vi "Etch-A-Sketch.vi"() -> ()   [LabVIEW 2017]
uses:
  Lockin/Lockin SR830.lvclass
  C:/LabVIEW-programs-dev/Instruments/Utility Classes/Readable/Readable.lvclass
  Wavelength meter/Wavelength Meter.lvclass
  Photon Counter/Photon Counter SR400.lvclass
  DAQ/DAQmx Analog.lvclass
  Power Meter/Power Meter.lvclass
  Fluke Multimeter/Fluke Multimeter.lvclass
  Cryostat/Cryostat.lvclass
  Utility Classes/Collection/Collection.lvclass
  <vilib>/Utility/file.llb/Write To Spreadsheet File (DBL).vi
  Main/Global/Misc.vi
  Main/Global/Flags.vi
  File IO/File IO.lvclass
  <vilib>/Analysis/NI_AALBase.lvlib
  Utility Classes/Readable/Readable.lvclass
panel:
  in  "Cryostat \nTemperature":bool
  in  "Fluke":bool
  out "Ave/Std Dev":dbl[](array[numeric])
  out "Average":dbl[](array[numeric])
  in  "Reset\nGraph":bool
  out "Y Range Extreme Value":dbl format="%#_4g"
  out "Latest Points":dbl[](array[numeric]) format="%#_5g"
  in  "Comments":string
  in  "Power Meter":bool
  out "Update Legend":bool
  in  "# of Points":i32=50 caption="Enter how many points to\nuse for Ave & Std Dev"
  out "Standard\nDeviation":dbl[](array[numeric])
  in  "Lockin \nSR810":bool
  in  "Lockin \nSR830":bool
  in  "Analog":bool
  in  "Photon \nCounter":bool
  in  "Wavelength \nMeter":bool
  in  "Graph Toggle":bool[](array[boolean])=[FALSE, FALSE, FALSE, FALSE, FALSE, FALSE, FALSE, FALSE, FALSE]
  in  "Display last":dbl[unit]=10.0
  in  "Time per point (s)":dbl[unit]=0.05 min=0.01 max=10.0
  in  "Start/Stop":bool
  out "XY Graph":T1(graph)
  in  "savedata?":bool
  in  "File Name":path
  in  "endprgm":bool
  # "<-- Select which instruments to use"
  # "Etch-A-Sketch"
  # "Don't\nSave"
  # "Save"
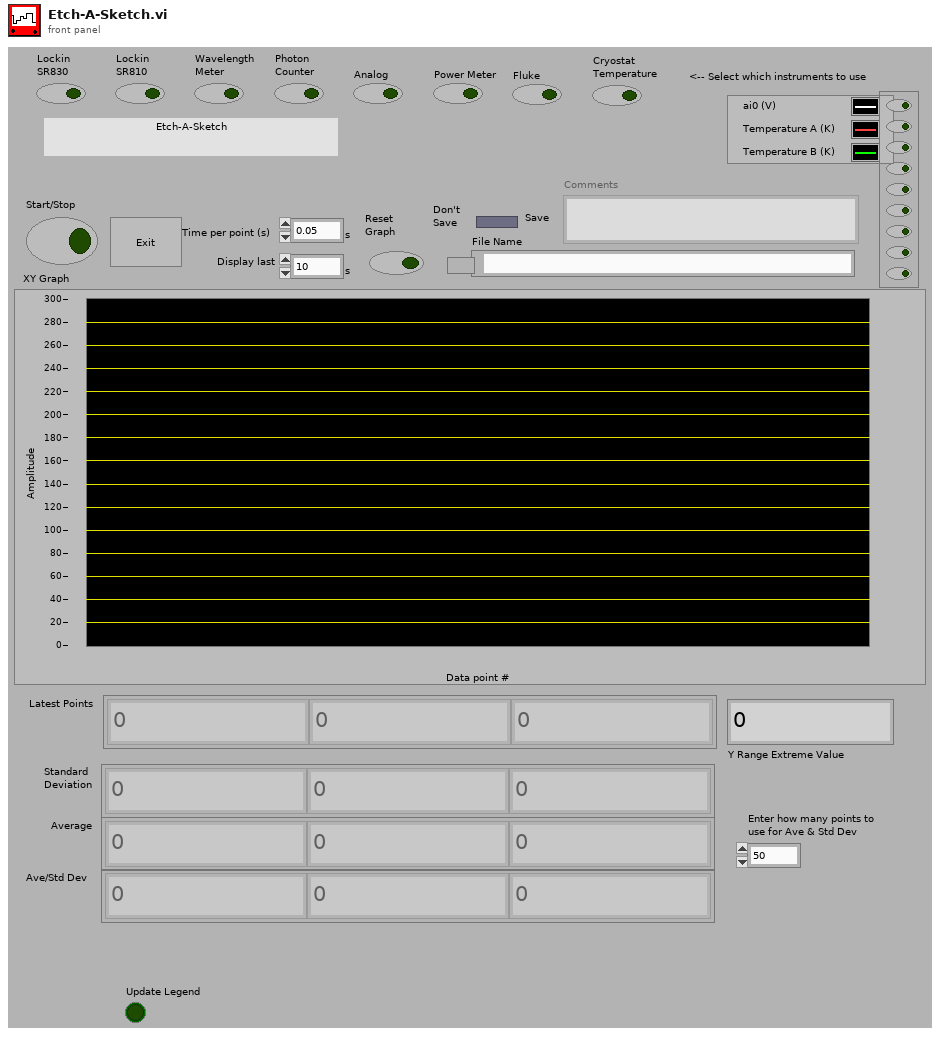
[diagram p1: front panel]
types:
  T1 = cluster{"Data Points":cluster{"t":timestamp, "x":dbl}[]}[]
  T2 = enum16{"open", "replace", "create", "open or create", "replace or create", "replace or create with confirmation"}
  T3 = typedef "Readable.lvclass/TX Graph.ctl" = cluster{"Data Points":cluster{"t":timestamp, "x":dbl}[]}[]
  T4 = typedef "Readable.lvclass/Channel Units.ctl" = string[]
  T5 = typedef "Readable.lvclass/Channel Names.ctl" = string[]
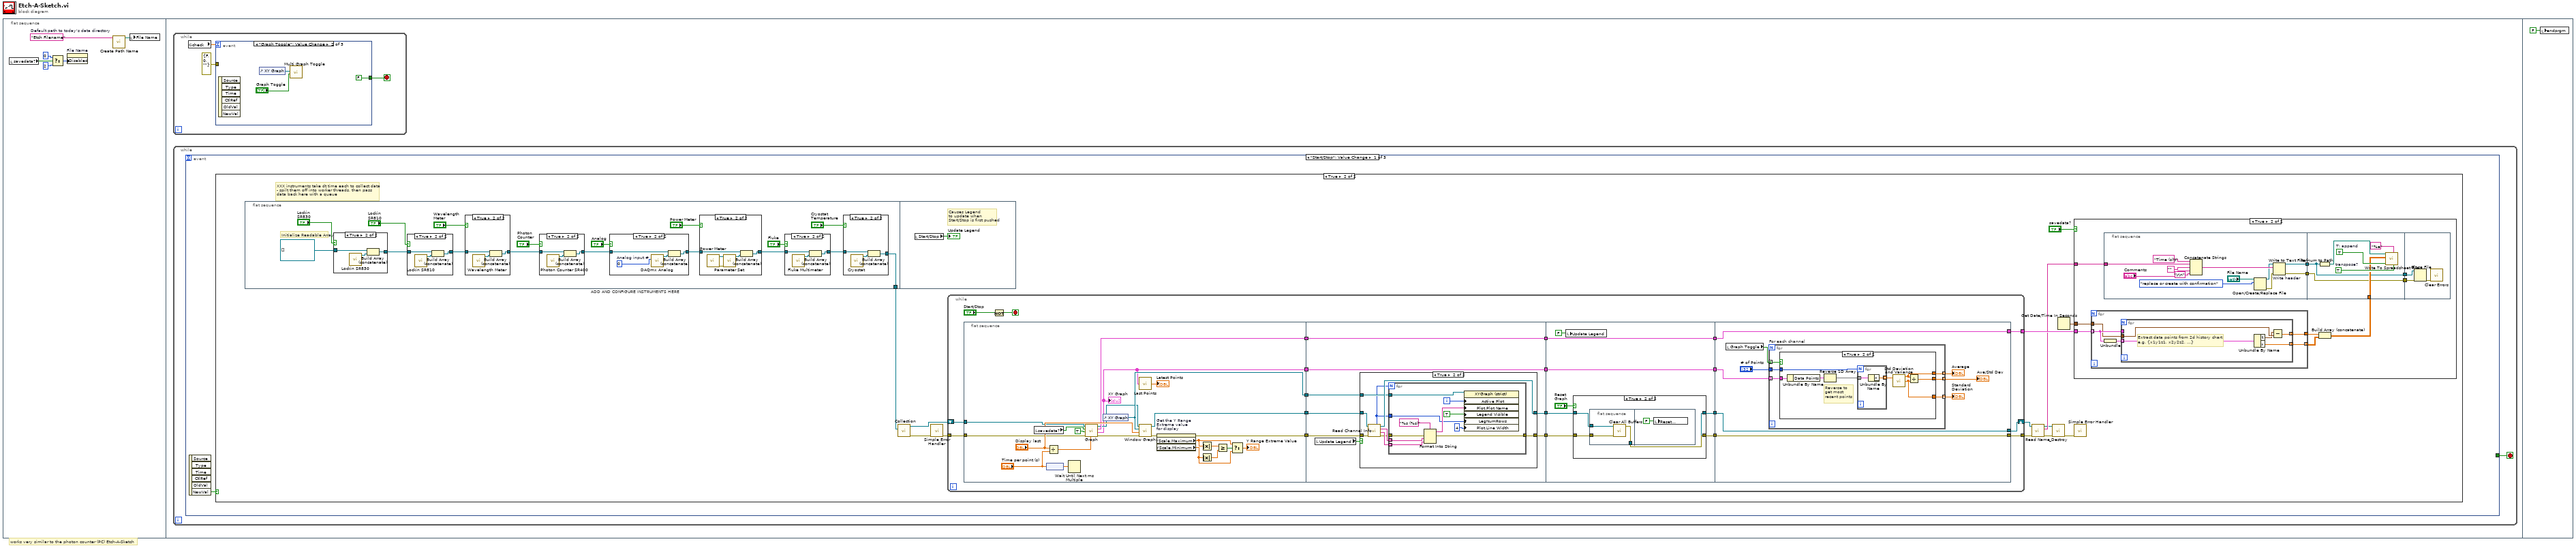
[diagram p0: block diagram]
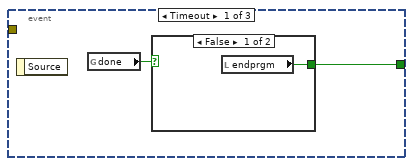
[diagram p2: hidden frame]
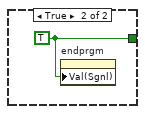
[diagram p3: hidden frame]
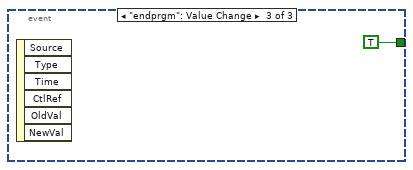
[diagram p4: hidden frame]
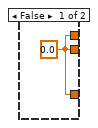
[diagram p9: hidden frame]
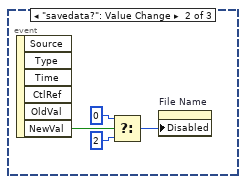
[diagram p18: hidden frame]
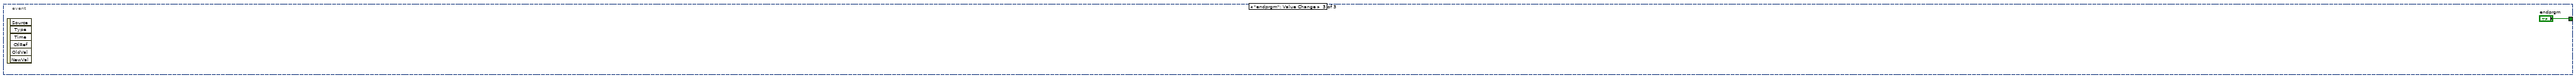
[diagram p19: hidden frame]
diagram:
  # "works very similar to the photon counter (PC) Etch-A-Sketch"
  n1 = flat-sequence {
    frame #0 {
      w1 = "Etch Filename"  # Default path to today's data directory
      n2 = local read "savedata?"() -> (w4:bool)
      n3 = Select(t=0, s=w4, f=2) -> (s? t:f=w3:i32)
      n4 = property on="File Name" class="Path"("Disabled"=w3) -> ()  [unwired: 2 in, 2 out]
      n5 = call "Create Path Name.vi"("filename"=w1) -> ("path"=w2:path)  [unwired: 1 in, 5 out]
      n6 = local write "File Name"(w2) -> ()
    }
    frame #1 {
      n7 = while {
        stop <- w9 stop-if-true
        n8 = global read "Misc.vi" "check"() -> (w8:dbl)
        n9 = event shown="[1] \"Graph Toggle\": Value Change" {
          selector: _ -> [_ _ _]
          dyn-events: _ -> [_ _ _]
          timeout: w8 -> [_ _ _]
          tunnel: [w10 FALSE TRUE] -> w9
          tunnel: errorcluster {"status"=FALSE, "code"=0, "source"=""} ("error out") -> [_ _ _]
          event Timeout {
            n10 = event-data() -> ()  [unwired: 2 out]
            n11 = global read "Flags.vi" "done"() -> (w11:bool)
            n12 = case shown="False" w11 {
              tunnel: [w12 w13] -> w10
              frame False {
                n13 = local read "endprgm"() -> (w12:bool)
              }
              frame True {
                w13 = TRUE
                n14 = property on="endprgm" class="Bool (strict)"("Val(Sgnl)"=w13) -> ()  [unwired: 2 in, 2 out]
              }
            }
          }
          event "Graph Toggle": Value Change {
            n15 = event-data() -> ()  [unwired: 7 out]
            n16 = control-ref of="XY Graph"() -> (w16:refnum<vi>)
            n17 = call "Multi Graph Toggle.vi"("Array"="Graph Toggle", "Waveform Chart"=w16) -> ()  [unwired: 1 in, 9 out]
          }
          event "endprgm": Value Change {
            n18 = event-data() -> ()  [unwired: 7 out]
          }
        }
      }
      n19 = while {
        stop <- w18 stop-if-true
        n20 = event shown="[0] \"Start/Stop\": Value Change" {
          selector: _ -> [_ _ _]
          dyn-events: _ -> [_ _ _]
          timeout: _ -> [_ _ _]
          tunnel: [_ _ "endprgm"] -> w18
          event "Start/Stop": Value Change {
            n21 = event-data() -> ("NewVal"=w19:bool)  [unwired: 6 out]
            n22 = case shown="True" w19 {
              frame False {
              }
              frame True {
                # "XXX instruments take dt time each to collect data\n- spilt them off into worker threads, then pass\ndata back here with a queue"
                n23 = flat-sequence "ADD AND CONFIGURE INSTRUMENTS HERE" {
                  tunnel: [w194] -> w20
                  frame #0 {
                    # "Initialize Readable Array"
                    n24 = case shown="True" "Lockin \nSR830" {
                      tunnel: refnum<class "Lockin SR830.lvclass">[] [] ("appended array") -> [w228 w230]
                      tunnel: [w228 w229] -> w206
                      frame False {
                      }
                      frame True {
                        n25 = call "Lockin SR830.vi"() -> ("Lockin SR830 out"=w231:refnum<class "Lockin SR830.lvclass">)  [unwired: 10 in, 1 out]
                        n26 = Build Array (concatenate)(w230, w231) -> (w229:refnum<class "Lockin SR830.lvclass">[])
                      }
                    }
                    n27 = case shown="True" "Lockin \nSR810" {
                      tunnel: w206 -> [w224 w227]
                      tunnel: [w224 w225] -> w205
                      frame False {
                      }
                      frame True {
                        n28 = call "Lockin SR810.vi"() -> ("Lockin SR830 out"=w226:refnum<class "Lockin SR830.lvclass">)  [unwired: 10 in, 1 out]
                        n29 = Build Array (concatenate)(w227, w226) -> (w225:refnum<class "Lockin SR830.lvclass">[])
                      }
                    }
                    n30 = case shown="True" "Wavelength \nMeter" {
                      tunnel: [w232 w234] -> w208
                      tunnel: w205 -> [w232 w233]
                      frame False {
                      }
                      frame True {
                        n31 = call "Wavelength Meter.vi"() -> ("Wavelength Meter out"=w235:refnum<class "Wavelength Meter.lvclass">)  [unwired: 1 in, 10 out]
                        n32 = Build Array (concatenate)(w233, w235) -> (w234:refnum<class "Readable.lvclass">[])
                      }
                    }
                    n33 = case shown="True" "Photon \nCounter" {
                      tunnel: [w236 w238] -> w209
                      tunnel: w208 -> [w236 w237]
                      frame False {
                      }
                      frame True {
                        n34 = call "Photon Counter SR400.vi"() -> ("Photon Counter SR400 out"=w239:refnum<class "Photon Counter SR400.lvclass">)  [unwired: 3 in, 8 out]
                        n35 = Build Array (concatenate)(w237, w239) -> (w238:refnum<class "Readable.lvclass">[])
                      }
                    }
                    n36 = case shown="True" "Analog" {
                      tunnel: w209 -> [w240 w242]
                      tunnel: [w240 w241] -> w198
                      frame False {
                      }
                      frame True {
                        w244 = u8 0  # Analog input #
                        n37 = call "DAQmx Analog.vi"("Analog input #"=w244) -> ("DAQmx Analog out"=w243:refnum<class "DAQmx Analog.lvclass">)  [unwired: 10 out]
                        n38 = Build Array (concatenate)(w242, w243) -> (w241:refnum<class "Readable.lvclass">[])
                      }
                    }
                    n39 = case shown="True" "Power Meter" {
                      tunnel: w198 -> [w218 w223]
                      tunnel: [w218 w222] -> w197
                      frame False {
                      }
                      frame True {
                        n40 = call "Power Meter.vi"() -> ("error out"=w219:errorcluster, "Power Meter out"=w221:refnum<class "Power Meter.lvclass">)  [unwired: 10 in]
                        n41 = call "Parameter Set.vi"("error in (no error)"=w219, "Power Meter in"=w221) -> ("Power Meter out"=w220:refnum<class "Power Meter.lvclass">)  [unwired: 8 in, 1 out]
                        n42 = Build Array (concatenate)(w223, w220) -> (w222:refnum<class "Readable.lvclass">[])
                      }
                    }
                    n43 = case shown="True" "Fluke" {
                      tunnel: w197 -> [w214 w217]
                      tunnel: [w214 w216] -> w195
                      frame False {
                      }
                      frame True {
                        n44 = call "Fluke Multimeter.vi"() -> ("Fluke Multimeter out"=w215:refnum<class "Fluke Multimeter.lvclass">)  [unwired: 10 in, 1 out]
                        n45 = Build Array (concatenate)(w217, w215) -> (w216:refnum<class "Readable.lvclass">[])
                      }
                    }
                    n46 = case shown="True" "Cryostat \nTemperature" {
                      tunnel: w195 -> [w210 w213]
                      tunnel: [w210 w212] -> w194
                      frame False {
                      }
                      frame True {
                        n47 = call "Cryostat.vi"() -> ("Cryostat out"=w211:refnum<class "Cryostat.lvclass">)  [unwired: 10 in, 1 out]
                        n48 = Build Array (concatenate)(w213, w211) -> (w212:refnum<class "Readable.lvclass">[])
                      }
                    }
                  }
                  frame #1 {
                    # "Causes Legend\nto update when\nStart/Stop is first pushed"
                    n49 = local read "Start/Stop"() -> (→"Update Legend":bool)
                  }
                }
                n50 = call "Collection.vi"("Array"=w20) -> ("error out"=w26:errorcluster, "Collection.lvclass out"=w27:refnum<class "Collection.lvclass">)  [unwired: 2 in, 7 out]
                n51 = call <vilib>:"Simple Error Handler.vi"("error in (no error)"=w26) -> ("error out"=w32:errorcluster)  [unwired: 1 in, 7 out]
                n52 = while {
                  shift-right: [w89] -> w31
                  shift-left: w27 -> [w91]
                  tunnel: w32 -> [w92]
                  tunnel: [w90] -> w29
                  tunnel: [w88] -> w21
                  stop <- w93 stop-if-true
                  n53 = flat-sequence {
                    tunnel: w92 -> [w112]
                    tunnel: w91 -> [w111]
                    tunnel: [w110] -> w87
                    tunnel: [w104] -> w86
                    tunnel: [w107] -> w85
                    tunnel: [w102] -> w84
                    tunnel: [w106] -> w83
                    tunnel: w87 -> [w119]
                    tunnel: [w119] -> w82
                    tunnel: w86 -> [w118]
                    tunnel: [w118] -> w81
                    tunnel: w85 -> [w125]
                    tunnel: w84 -> [w124]
                    tunnel: w83 -> [w123]
                    tunnel: [w121] -> w80
                    tunnel: [w120] -> w79
                    tunnel: w82 -> [w149]
                    tunnel: [w149] -> w78
                    tunnel: [w153] -> w77
                    tunnel: [w151] -> w76
                    tunnel: w81 -> [w148]
                    tunnel: [w148] -> w75
                    tunnel: w80 -> [w154]
                    tunnel: w79 -> [w152]
                    tunnel: [w172] -> w90
                    tunnel: w78 -> [w172]
                    tunnel: [w171] -> w89
                    tunnel: w77 -> [w171]
                    tunnel: [w170] -> w88
                    tunnel: w76 -> [w170]
                    tunnel: w75 -> [w175]
                    frame #0 {
                      n54 = local read "savedata?"() -> (w113:bool)
                      n55 = node("Time per point (s)") -> (w108:dbl)
                      n56 = Divide(x="Display last", y="Time per point (s)") -> (x/y=w115:dbl)
                      n57 = Wait Until Next ms Multiple(millisecond multiple=w108) -> ()  [unwired: 1 out]
                      n58 = call-dynamic "Graph.vi"("Ring size (points) (1024)"=w115, "error in (no error)"=w112, "Store Ring? (f)"=TRUE, "Store History? (f)"=w113, "Collection in"=w111) -> ("error out"=w116:errorcluster, "Ring Buffers"=w104:T3, "History Buffers"=w110:T3, "Collection out"=w105:refnum<class "Collection.lvclass">)  [unwired: 3 out]
                      "XY Graph" <- w104
                      n59 = control-ref of="XY Graph"() -> (w107:refnum<vi>)
                      n60 = call "Last Points.vi"("Ring Buffers"=w104) -> ("Latest Points"=→"Latest Points":dbl[])
                      n61 = call-dynamic "Window Graph.vi"("error in (no error)"=w116, "Window"="Display last", "Graph ref"=w107, "Readable in"=w105) -> ("error out"=w101:errorcluster, "Readable out"=w106:refnum<class "Collection.lvclass">)  [unwired: 6 in]
                      n62 = property on="Get the Y Range\nExtreme value\nfor display" class="XYGraph (strict)"(error in=w101) -> (error out=w102:errorcluster, "YScale.Maximum"=w97:dbl, "YScale.Minimum"=w96:dbl)  [unwired: 1 in, 1 out]
                      n63 = Absolute Value(x=w97) -> (abs(x)=w100:dbl)
                      n64 = Absolute Value(x=w96) -> (abs(x)=w99:dbl)
                      n65 = Greater Or Equal?(x=w100, y=w99) -> (x >= y?=w98:bool)
                      n66 = Select(t=w97, s=w98, f=w96) -> (s? t:f=→"Y Range Extreme Value":dbl)
                    }
                    frame #1 {
                      n67 = local read "Update Legend"() -> (w122:bool)
                      n68 = case shown="True" w122 {
                        tunnel: w123 -> [w126 w136]
                        tunnel: [w126 w135] -> w121
                        tunnel: w124 -> [w127 w132]
                        tunnel: [w127 w130] -> w120
                        tunnel: w125 -> [_ w129]
                        frame False {
                        }
                        frame True {
                          n69 = call "Read Channel Info.vi"("error in (no error)"=w132, "Readable.lvclass in"=w136) -> ("error out"=w131:errorcluster, "Channel Units"=w133:T4, "Channel Names"=w134:T5, "Readable.lvclass out"=w135:refnum<class "Collection.lvclass">, "#Channels"=w128:i32)  [unwired: 5 in]
                          n70 = for {
                            N: w128 -> [_]
                            tunnel: w134 -> [w144] mode=indexing
                            tunnel: w131 -> [w146]
                            tunnel: w133 -> [w143] mode=indexing
                            tunnel: [w141] -> w130
                            tunnel: w129 -> [w140]
                            tunnel: w128 -> [w138]
                            i -> [w147]
                            n71 = Format Into String(format string="%s (%s)", error in=w146, w144, w143) -> (resulting string=w142:string, error out=w141:errorcluster)  [unwired: 1 in]
                            n72 = property on="Property Node" class="XYGraph (strict)"(reference=w140, "Active Plot"=w147, "Plot.Plot Name"=w142, "Legend Visible"=TRUE ("Legend:Visible"), "LegNumRows"=w138, "Plot.Line Width"=u32 4 ("x")) -> ()  [unwired: 1 in, 2 out]
                          }
                        }
                      }
                    }
                    frame #2 {
                      n73 = local write "Update Legend"(FALSE ("Update Legend")) -> ()
                      n74 = case shown="True" "Reset\nGraph" {
                        tunnel: w154 -> [w157 w161]
                        tunnel: [w157 w158] -> w153
                        tunnel: w152 -> [w156 w160]
                        tunnel: [w156 w159] -> w151
                        frame False {
                        }
                        frame True {
                          n75 = flat-sequence {
                            tunnel: w161 -> [w165]
                            tunnel: w160 -> [w164]
                            tunnel: [w163] -> w159
                            tunnel: [w162] -> w158
                            frame #0 {
                              n76 = call "Clear All Buffers.vi"("error in (no error)"=w164, "Collection.lvclass In"=w165) -> ("error Out"=w163:errorcluster, "Collection.lvclass Out"=w162:refnum<class "Collection.lvclass">)  [unwired: 8 in]
                            }
                            frame #1 {
                              n77 = local write "Reset\nGraph"(FALSE ("Clear")) -> ()
                            }
                          }
                        }
                      }
                    }
                    frame #3 {
                      n78 = local read "Graph Toggle"() -> (w167:bool[])
                      n79 = for "For each channel" {
                        tunnel: w175 -> [w181] mode=indexing
                        tunnel: "# of Points" -> [w180]
                        tunnel: [w179] -> w173 mode=indexing
                        tunnel: w167 -> [w178] mode=indexing
                        tunnel: [w177] -> w169 mode=indexing
                        tunnel: [w176] -> w168 mode=indexing
                        n80 = case shown="True" w178 {
                          tunnel: w181 -> [_ w190]
                          tunnel: w180 -> [_ w187]
                          tunnel: [w182 w186] -> w179
                          tunnel: [w182 w183] -> w177
                          tunnel: [w182 w185] -> w176
                          frame False {
                            w182 = 0.0 ("standard deviation")
                          }
                          frame True {
                            # "Reverse to\nget most \nrecent points"
                            n81 = Unbundle By Name(w190) -> ("Data Points"=w189:cluster{"t":timestamp, "x":dbl}[])
                            n82 = Reverse 1D Array(array=w189) -> (reversed array=w188:cluster{"t":timestamp, "x":dbl}[])
                            n83 = for {
                              N: w187 -> [_]
                              tunnel: w188 -> [w192] mode=indexing
                              tunnel: [w191] -> w184 mode=indexing
                              n84 = Unbundle By Name(w192) -> ("x"=w191:dbl)
                            }
                            n85 = call <vilib>:"Std Deviation and Variance.vi"("X"=w184) -> ("mean"=w183:dbl, "standard deviation"=w186:dbl)  [unwired: 1 in, 1 out]
                            n86 = Divide(x=w183, y=w186) -> (x/y=w185:dbl)
                          }
                        }
                      }
                      "Standard\nDeviation" <- w173
                      "Average" <- w169
                      "Ave/Std Dev" <- w168
                    }
                  }
                  n87 = Not(x="Start/Stop") -> (.not. x?=w93:bool)
                }
                n88 = call-dynamic "Read Name.vi"("error in (no error)"=w21, "Instrument.lvclass in"=w31) -> ("error out"=w22:errorcluster, "Name"=w25:string, "Instrument.lvclass out"=w24:refnum<class "Collection.lvclass">)  [unwired: 7 out]
                n89 = call-dynamic "_Destroy.vi"("error in (no error)"=w22, "Collection in"=w24) -> ("error out"=w23:errorcluster)  [unwired: 9 out]
                n90 = Get Date/Time In Seconds() -> (seconds since 1Jan1904=w28:timestamp)
                n91 = case shown="True" "savedata?" {
                  tunnel: w25 -> [_ w38]
                  tunnel: w29 -> [_ w37]
                  tunnel: w28 -> [_ w36]
                  frame False {
                  }
                  frame True {
                    n92 = for {
                      tunnel: w37 -> [w68] mode=indexing
                      tunnel: [w69] -> w33 mode=indexing
                      tunnel: [w66] -> w35
                      tunnel: w36 -> [w65]
                      n93 = Unbundle(w68) -> ("Data Points"=w67:cluster{"t":timestamp, "x":dbl}[])
                      n94 = for {
                        tunnel: [w73] -> w69 mode=indexing
                        tunnel: w68 -> [_]
                        tunnel: w67 -> [w74] mode=indexing
                        tunnel: [w70] -> w66 mode=indexing
                        tunnel: w65 -> [w72]
                        # "Extract data points from 2d history chart \ne.g. {x1y1z1, x2y2z2, ...}"
                        n95 = Unbundle By Name(w74) -> ("t"=w71:timestamp, "x"=w73:dbl)
                        n96 = Subtract(x=w71, y=w72) -> (x-y=w70:dbl)
                      }
                    }
                    n97 = flat-sequence {
                      tunnel: [w53] -> w41
                      tunnel: [w50] -> w39
                      tunnel: w38 -> [w51]
                      tunnel: [w57] -> w42
                      tunnel: w41 -> [w57]
                      tunnel: w34 -> [w59]
                      tunnel: [w55] -> w40
                      tunnel: w39 -> [w55]
                      tunnel: w42 -> [w64]
                      tunnel: w40 -> [w63]
                      frame #0 {
                        n98 = Concatenate Strings("Time (s)\t" ("string"), w51, "", "Comments", "\r\n") -> (w48:string)
                        n99 = Open/Create/Replace File(file path (use dialog)="File Name", operation (0:open)=T2."replace or create with confirmation") -> (refnum out=w46:refnum<file>, error out=w49:errorcluster)  [unwired: 1 in, 4 out]
                        n100 = Write to Text File "Write header"(file (use dialog)=w46, text=w48, error in=w49) -> (refnum out=w53:refnum<file>, error out=w50:errorcluster)  [unwired: 2 out]
                      }
                      frame #1 {
                        w60 = TRUE  # transpose?
                        w61 = TRUE  # T: append
                        n101 = Refnum to Path(1:w57) -> (0:w56:path)
                        n102 = call-poly <vilib>:"Write To Spreadsheet File.vi"("transpose? (no:F)"=w60, "format (%.3f)"="%e", "append to file? (new file:F)"=w61, "2D data"=w59, "file path (dialog if empty)"=w56) -> ()  [unwired: 1 in, 3 out]
                      }
                      frame #2 {
                        n103 = Close File(refnum=w64, error in=w63) -> (error out=w62:errorcluster)  [unwired: 1 out]
                        n104 = call <vilib>:"Clear Errors.vi"("error in (no error)"=w62) -> ()  [unwired: 1 in, 6 out]
                      }
                    }
                    n105 = Build Array (concatenate)(w35, w33) -> (w34:dbl[][])
                  }
                }
                n106 = call <vilib>:"Simple Error Handler.vi"("error in (no error)"=w23) -> ()  [unwired: 1 in, 8 out]
              }
            }
          }
          event "savedata?": Value Change {
            n107 = event-data() -> ("NewVal"=w249:bool)  [unwired: 6 out]
            n108 = Select(t=0, s=w249, f=2) -> (s? t:f=w246:i32)
            n109 = property on="File Name" class="Path"("Disabled"=w246) -> ()  [unwired: 2 in, 2 out]
          }
          event "endprgm": Value Change {
            n110 = event-data() -> ()  [unwired: 7 out]
          }
        }
      }
    }
    frame #2 {
      n111 = local write "endprgm"(FALSE) -> ()
    }
  }
